vi "Waveform_Extract from Start and End time.vi"(8 "Error":errorcluster, 9 "End Time":dbl, 10 "Begin Time":dbl, 11 "Waveform":T1) -> (0 "Error Out":errorcluster, 1 "End Index Out":i32, 2 "Start Index Out":i32, 3 "Waveform Out":T1)   [LabVIEW 2015]
doc: "Retrieves a subset of a waveform at a specified time or index. You must manually select the polymorphic instance you want to use."
uses:
  Universal Controls/Waveform_Data.ctl
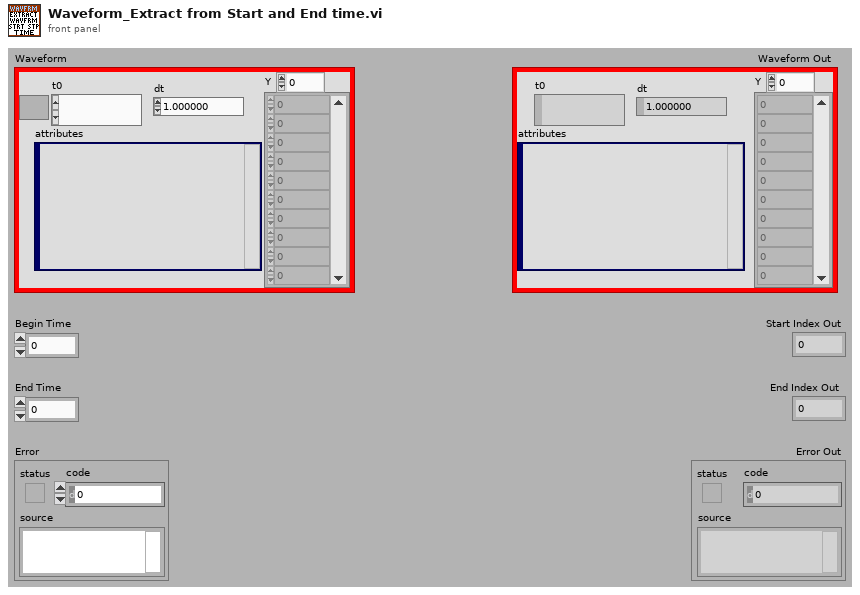
[diagram p1: front panel]
types:
  T1 = typedef "Waveform_Data.ctl" = waveform(dbl)
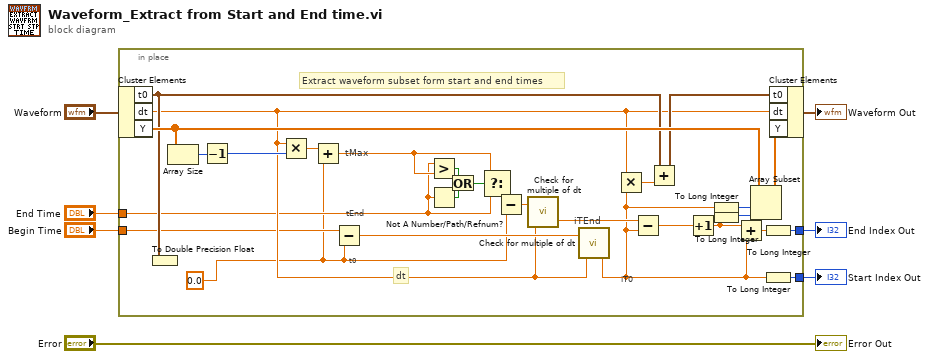
[diagram p0: block diagram]
diagram:
  n1 = in-place {
    in-place-border: "Begin Time" -> [w10]
    in-place-border: "End Time" -> [w9]
    in-place-border: [w24] -> w5
    in-place-border: [w23] -> w4
    w8 = 0.0 ("double precision float")
    # "Extract waveform subset form start and end times"
    # "dt"
    # "iTEnd"
    # "iT0"
    # "tEnd"
    # "t0"
    # "tMax"
    n2 = in-place-cluster #1("Waveform") -> ("t0"=w13:timestamp, "dt"=w11:dbl, "Y"=w15:dbl[])
    n3 = To Double Precision Float(number=w13) -> ()  [unwired: 1 out]
    n4 = Array Size(array=w15) -> (size(s)=w33:i32)
    n5 = Decrement(x=w33) -> (x-1=w32:i32)
    n6 = Multiply(x=w11, y=w32) -> (x*y=w35:dbl)
    n7 = Add(x=w35, y=w8) -> (x+y=w34:dbl)
    n8 = Subtract(x=w10, y=w8) -> (x-y=w28:dbl)
    n9 = Greater?(x=w9, y=w34) -> (0:w31:bool)
    n10 = Not A Number/Path/Refnum?(number/path/refnum=w9) -> (NaN/Path/Refnum?=w30:bool)
    n11 = Or(x=w31, y=w30) -> (x .or. y?=w29:bool)
    n12 = Select(t=w34, s=w29, f=w9) -> (s? t:f=w26:dbl)
    n13 = Subtract(x=w26, y=w8) -> (x-y=w27:dbl)
    n14 = call <vilib>:"Check for multiple of dt.vi"("dt"=w11, "time"=w27) -> ("iQuotient"=w25:dbl)  [unwired: 1 out]
    n15 = call <vilib>:"Check for multiple of dt.vi"("dt"=w11, "time"=w28) -> ("iQuotient"=w20:dbl)  [unwired: 1 out]
    n16 = Multiply(x=w11, y=w20) -> (x*y=w18:dbl)
    n17 = Subtract(x=w25, y=w20) -> (x-y=w22:dbl)
    n18 = Add(x=w13, y=w18) -> (x+y=w12:timestamp)
    n19 = Increment(x=w22) -> (x+1=w21:dbl)
    n20 = To Long Integer(number=w20) -> (32bit integer=w16:i32)
    n21 = To Long Integer(number=w21) -> (32bit integer=w17:i32)
    n22 = Add(x=w21, y=w20) -> (x+y=w19:dbl)
    n23 = Array Subset(array=w15, index=w16, length=w17) -> (w14:dbl[])
    n24 = To Long Integer(number=w19) -> (32bit integer=w23:i32)
    n25 = To Long Integer(number=w20) -> (32bit integer=w24:i32)
    n26 = in-place-cluster #1("t0"=w12, "dt"=w11, "Y"=w14) -> (→"Waveform Out":T1)
  }
  "Start Index Out" <- w5
  "End Index Out" <- w4
  "Error Out" <- "Error"
